vi "if strike.vi"(8 "error in (no error)":errorcluster, 11 "KNR in":T2) -> (0 "error out":errorcluster, 3 "KNR out":T2, 4 "is strike?":bool=TRUE)   [LabVIEW 2013]
uses:
  <userlib>/KNR OS 3.0 LabVIEW Toolkit/Type Definition/KNR3 Reference.ctl
  <userlib>/_FPGA Interface Advanced Tools/FPGA Interface Base/FPGA Interface Base.lvclass
  <userlib>/KNR OS 3.0 LabVIEW Toolkit/Type Definition/Resource.ctl
panel:
  out "?":T1(plugin-control)
  out "?":T1(plugin-control)
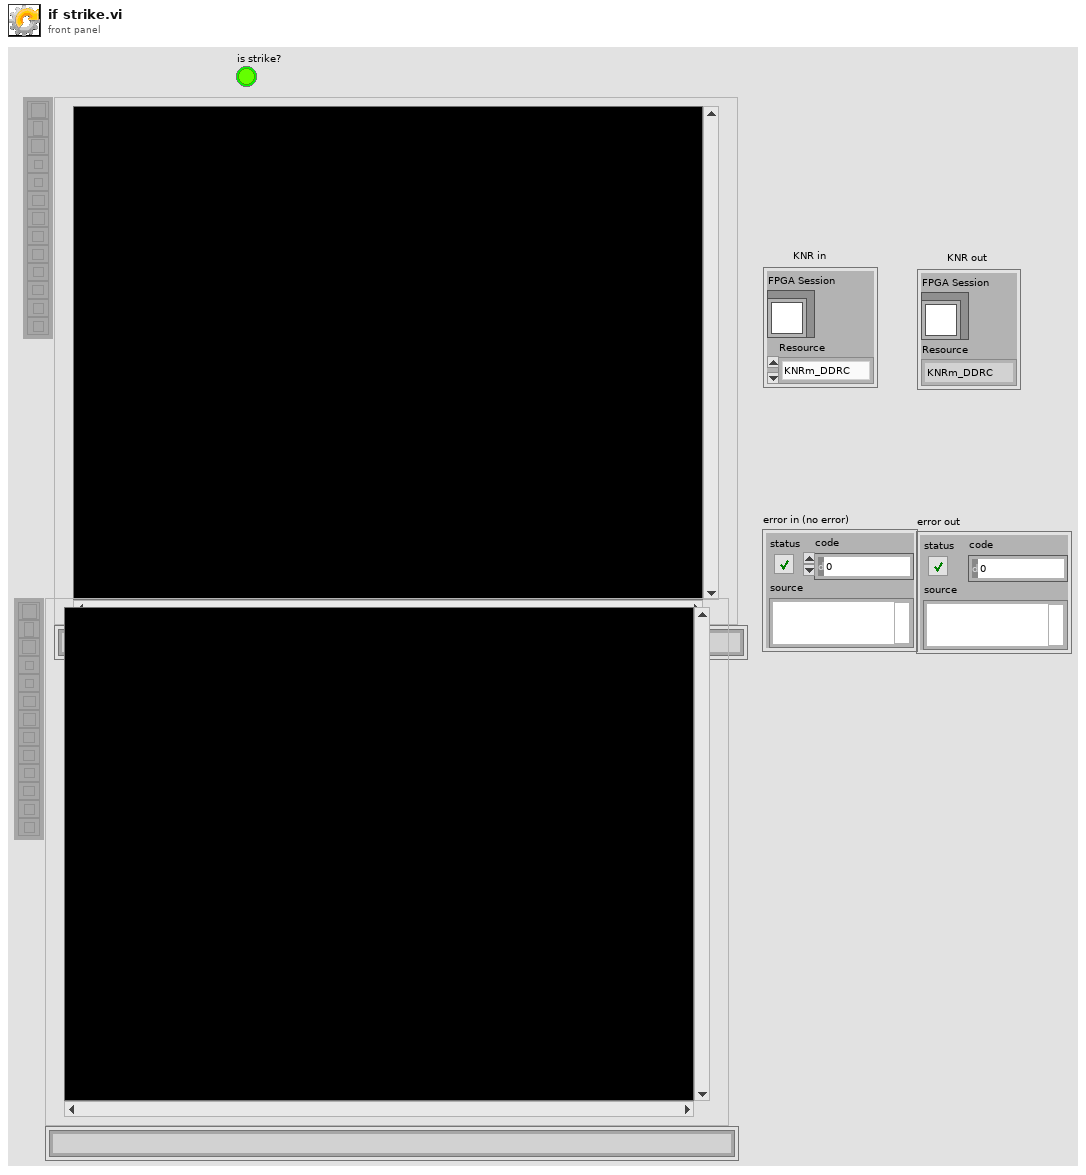
[diagram p1: front panel]
types:
  T1 = typedef "IMAQ Image.ctl" = refnum<image>
  T2 = typedef "KNR3 Reference.ctl" = cluster{"FPGA Session":refnum<class "FPGA Interface Base.lvclass">, "Resource":T3}
  T3 = typedef "Resource.ctl" = enum16{"KNRm_DDRC", "KNRm_DDDD", "KNRm_DDDR", "KNRm_DDDC", "KNR"}
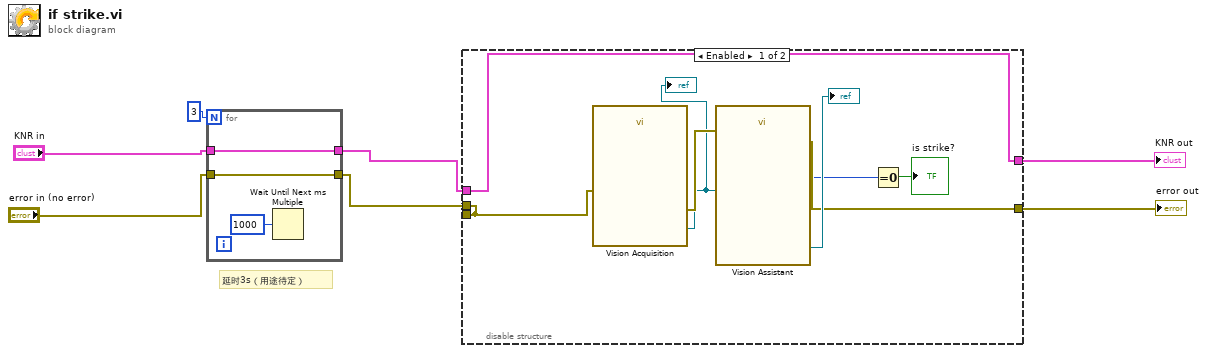
[diagram p0: block diagram]
diagram:
  # "延时3s（用途待定）"
  n1 = for {
    N: 3 -> [_]
    tunnel: "KNR in" -> [w9]
    tunnel: "error in (no error)" -> [w10]
    tunnel: [w10] -> w3
    tunnel: [w9] -> w4
    n2 = Wait Until Next ms Multiple(millisecond multiple=u32 1000) -> ()  [unwired: 1 out]
  }
  n3 = disable-structure shown="Enabled" {
    disable-tunnel: [w17 _] -> w7
    disable-tunnel: [w13 _] -> w6
    disable-tunnel: [w12 _] -> _
    disable-tunnel: w4 -> [w13 _]
    disable-tunnel: w3 -> [w12 _]
    frame Enabled {
      n4 = call "Vision Acquisition"("error in"=w12) -> ("Image Out"=w11:T1, "error out"=w16:errorcluster)  [unwired: 25 in]
      "?" <- w11
      n5 = call "Vision Assistant"("Image In"=w11, "error in"=w16) -> ("Image Out"=→"?":T1, "Number of Particles (Particle Analysis 1)"=w15:i32, "error out"=w17:errorcluster)  [unwired: 23 in]
      n6 = Equal To 0?(x=w15) -> (x = 0?=→"is strike?":bool)
    }
    frame Disabled {
    }
  }
  "error out" <- w7
  "KNR out" <- w6
